vi "Create Name.vi"(6 "Name":string, 8 "error in":errorcluster, 9 "Name Library File Path":path, 10 "Active Project":refnum<vi>) -> (0 "error out":errorcluster, 2 "Name":T1)   [LabVIEW 2020, in "_Rescript.lvlib" / "Actor.lvlib" / "Actor.lvclass"]
uses:
  Actor.lvclass
  Name.ctl
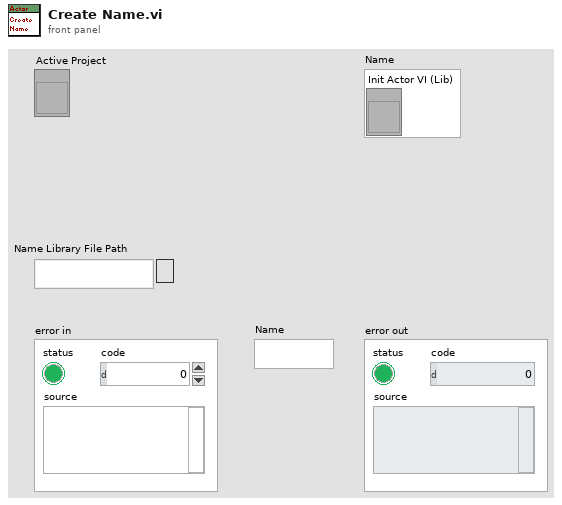
[diagram p1: front panel]
types:
  T1 = typedef "_Rescript.lvlib/Actor.lvlib/Actor.lvclass/Name.ctl" = cluster{"Init Actor VI (Lib)":refnum<vi>}
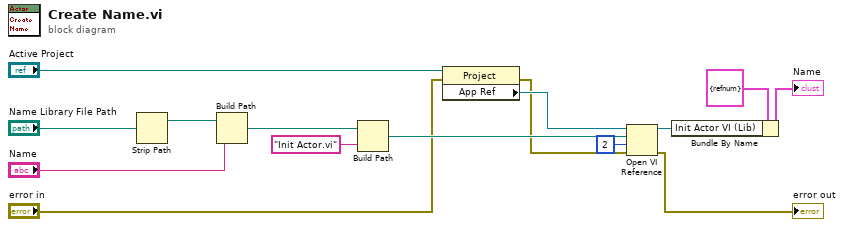
[diagram p0: block diagram]
diagram:
  n1 = Strip Path(path="Name Library File Path") -> (stripped path=w15:path)  [unwired: 1 out]
  n2 = Build Path(base path=w15, name or relative path="Name") -> (appended path=w14:path)
  n3 = Build Path(base path=w14, name or relative path="Init Actor.vi" ("format string")) -> (appended path=w10:path)
  n4 = property class="Project"(reference="Active Project", error in="error in") -> (error out=w1:errorcluster, "App Ref"=w11:refnum<vi>)  [unwired: 1 out]
  n5 = Open VI Reference(application reference (local)=w11, vi path=w10, options=2, error in (no error)=w1) -> (vi reference=w9:refnum<vi>, error out=→"error out":errorcluster)  [unwired: 2 in]
  n6 = Bundle By Name(cluster=T1 {"Init Actor VI (Lib)"=refnum} ("Name"), "Init Actor VI (Lib)"=w9) -> (→"Name":T1)
